vi "Overlay Straight Edges.vi"(6 "All Edges (Pixel)":cluster{"Edge Information":T1[]}[](array[cluster]) {"Edge Information"."Distance (Real-World)" format="%.2f"; "Edge Information"."Location (Real-World)"."Y" format="%.2f"; "Edge Information"."Location (Real-World)"."X" format="%.2f"; "Edge Information"."Noise" format="%.2f"; "Edge Information"."Location (Pixel)"."Y" format="%.2f"; "Edge Information"."Location (Pixel)"."X" format="%.2f"; "Edge Information"."Strength" format="%.2f"; "Edge Information"."Distance (Pixel)" format="%.2f"}, 8 "error in":errorcluster, 9 "Search Lines Information":T2(array[cluster]) {"Edges"."Distance (Real-World)" format="%.2f"; "Edges"."Location (Real-World)"."Y" format="%.2f"; "Edges"."Location (Real-World)"."X" format="%.2f"; "Edges"."Noise" format="%.2f"; "Edges"."Location (Pixel)"."Y" format="%.2f"; "Edges"."Location (Pixel)"."X" format="%.2f"; "Edges"."Strength" format="%.2f"; "Edges"."Distance (Pixel)" format="%.2f"; "End Point"."Y" format="%.2f"; "End Point"."X" format="%.2f"; "Start Point"."Y" format="%.2f"; "Start Point"."X" format="%.2f"}, 10 "Straight Edges":T4(array[cluster]) {"Point2 (Real-World)"."Y" format="%.2f"; "Point2 (Real-World)"."X" format="%.2f"; "Point1 (Real-World)"."Y" format="%.2f"; "Point1 (Real-World)"."X" format="%.2f"; "Point2 (Pixels)"."Y" format="%.2f"; "Point2 (Pixels)"."X" format="%.2f"; "Point1 (Pixels)"."Y" format="%.2f"; "Point1 (Pixels)"."X" format="%.2f"}, 11 "Image In":T3) -> (0 "error out":errorcluster, 3 "Image Out":T3)   [LabVIEW 2015]
doc: "Overlays multiple lines on the image using the results from the Find Straight Edge function."
uses:
  <vilib>/vision/Image Controls.llb/IMAQ Image.ctl
  <vilib>/vision/Measure.llb/Edge New.ctl
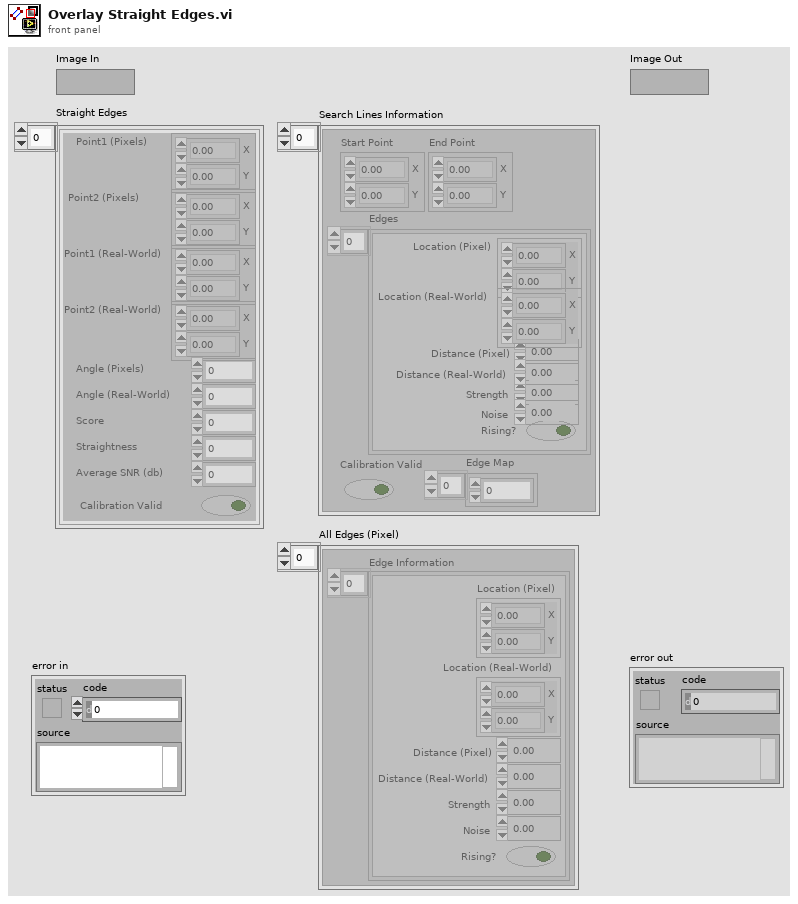
[diagram p1: front panel]
types:
  T1 = typedef "Edge New.ctl" = cluster{"Location (Pixel)":cluster{"X":sgl, "Y":sgl}, "Location (Real-World)":cluster{"X":sgl, "Y":sgl}, "Distance (Pixel)":dbl, "Distance (Real-World)":dbl, "Strength":dbl, "Noise":dbl, "Rising?":bool}
  T2 = cluster{"Start Point":cluster{"X":sgl, "Y":sgl}, "End Point":cluster{"X":sgl, "Y":sgl}, "Edges":T1[], "Edge Map":dbl[], "Calibration Valid":bool}[]
  T3 = typedef "IMAQ Image.ctl" = refnum<image>
  T4 = cluster{"Point1 (Pixels)":cluster{"X":sgl, "Y":sgl}, "Point2 (Pixels)":cluster{"X":sgl, "Y":sgl}, "Point1 (Real-World)":cluster{"X":sgl, "Y":sgl}, "Point2 (Real-World)":cluster{"X":sgl, "Y":sgl}, "Angle (Pixels)":dbl, "Angle (Real-World)":dbl, "Score":dbl, "Straightness":dbl, "Average SNR (db)":dbl, "Calibration Valid":bool}[]
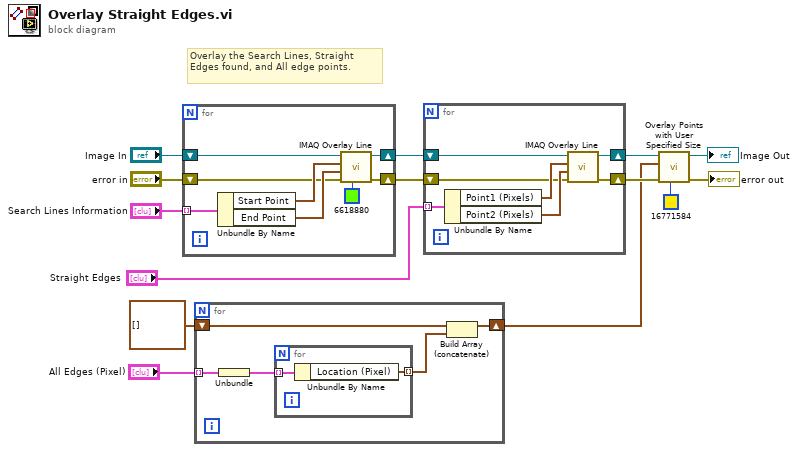
[diagram p0: block diagram]
diagram:
  # "Overlay the Search Lines, Straight Edges found, and All edge points."
  n1 = for {
    shift-right: [w21] -> w9
    shift-left: "Image In" -> [w22]
    tunnel: "Search Lines Information" -> [w20] mode=indexing
    shift-right: [w16] -> w10
    shift-left: "error in" -> [w17]
    n2 = Unbundle By Name(w20) -> ("Start Point"=w19:cluster{"X":sgl, "Y":sgl}, "End Point"=w18:cluster{"X":sgl, "Y":sgl})
    n3 = call "IMAQ Overlay Line"("Color"=u32 6618880, "error in (no error)"=w17, "End Point"=w18, "Start Point"=w19, "Image"=w22) -> ("error out"=w16:errorcluster, "Image Out"=w21:T3)  [unwired: 5 in]
  }
  n4 = for {
    tunnel: "All Edges (Pixel)" -> [w27] mode=indexing
    shift-right: [w24] -> w4
    shift-left: cluster{"X":sgl, "Y":sgl}[] [] -> [w23]
    n5 = Unbundle(w27) -> ("Edge Information"=w26:T1[])
    n6 = for {
      tunnel: w26 -> [w29] mode=indexing
      tunnel: [w28] -> w25 mode=indexing
      n7 = Unbundle By Name(w29) -> ("Location (Pixel)"=w28:cluster{"X":sgl, "Y":sgl})
    }
    n8 = Build Array (concatenate)(w23, w25) -> (w24:cluster{"X":sgl, "Y":sgl}[])
  }
  n9 = for {
    shift-right: [w35] -> w6
    shift-left: w9 -> [w36]
    tunnel: "Straight Edges" -> [w34] mode=indexing
    shift-right: [w30] -> w5
    shift-left: w10 -> [w31]
    n10 = Unbundle By Name(w34) -> ("Point1 (Pixels)"=w33:cluster{"X":sgl, "Y":sgl}, "Point2 (Pixels)"=w32:cluster{"X":sgl, "Y":sgl})
    n11 = call "IMAQ Overlay Line"("error in (no error)"=w31, "End Point"=w32, "Start Point"=w33, "Image"=w36) -> ("error out"=w30:errorcluster, "Image Out"=w35:T3)  [unwired: 6 in]
  }
  n12 = call "Overlay Points with User Specified Size.vi"("Color"=u32 16771584, "error in"=w5, "Points"=w4, "Image In"=w6) -> ("error out"=→"error out":errorcluster, "Image Out"=→"Image Out":T3)  [unwired: 6 in]
